vi "Store Configuration Parameters.vi"(8 "error in (no error)":errorcluster, 10 "refnum":T1, 11 "VacuumLine Configuration in":refnum<class "VacuumLine Configuration.lvclass">) -> (0 "error out":errorcluster, 2 "refnum out":T1, 3 "VacuumLine Configuration out":refnum<class "VacuumLine Configuration.lvclass">)   [LabVIEW 2016, in "Hardware.lvlib" / "VacuumLine.lvlib" / "VacuumLine Configuration.lvclass"]
uses:
  <userlib>/Common Components/Hardware/Abstract System/VacuumLine/VacuumLine Config/VacuumLine Configuration.lvclass
  <vilib>/Utility/config.llb/Config Data RefNum.ctl
  <userlib>/Common Components/Hardware/Abstract System/VacuumLine/VacuumLine Config/VacuumLine Configuration.lvclass/VacuumLine Configuration.ctl
  <userlib>/Common Components/Hardware/Abstract System/VacuumLine/VacuumLine/VacuumLine.lvclass/VacuumLine.ctl
  <userlib>/Common Components/Hardware/Abstract System/VacuumLine/VacuumLine/Read VacuumLine Params.vi
  <userlib>/Common Components/Hardware/Abstract System/VacuumLine/VacuumLine/Read Array of Move Button Configurations.vi
  <userlib>/Configuration Dialog Actor/Configuration.lvclass
  <userlib>/Common Components/Hardware/Motor/Motor Config/Motor Configuration.lvclass
  <vilib>/Utility/config.llb/NI_LVConfig.lvlib
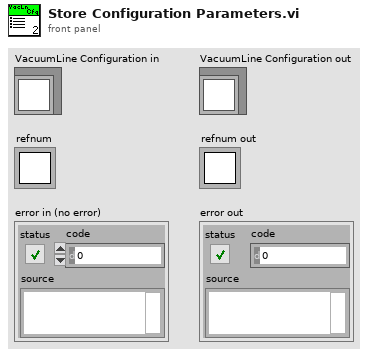
[diagram p1: front panel]
types:
  T1 = typedef "NI_LVConfig.lvlib/Config Data RefNum.ctl" = refnum<k1>
  T2 = typedef "Hardware.lvlib/VacuumLine.lvlib/VacuumLine.lvclass/VacuumLine Params.ctl" = cluster{"Motion Limits":cluster{"min":dbl, "max":dbl}, "No. of Conflict Zones":u8, "Conflict Zones (mm)":cluster{"with":string, "from":dbl, "to":dbl, "buffer":dbl}[], "Valve Complexes":T3[], "max( |Motor Pos - LRF Distance| )":dbl}
  T3 = typedef "Hardware.lvlib/VacuumLine.lvlib/VacuumLine.lvclass/Valve Complex.ctl" = cluster{"LogicIO Module":string, "Valve Open":T4, "Optical Switch -":T4, "Optical Switch +":T4, "Valve Closed Status Alert":cluster{"Pin#":u8, "Option":enum16{"Not Used", "Normally Closed"}}}
  T4 = typedef "Hardware.lvlib/VacuumLine.lvlib/VacuumLine.lvclass/Logic Cluster.ctl" = cluster{"Pin#":u8, "Location":dbl, "Tolerance":dbl}
  T5 = typedef "Hardware.lvlib/VacuumLine.lvlib/VacuumLine.lvclass/Button Config Cluster.ctl" = cluster{"Enabled?":bool, "Text on button":string, "Target pos":dbl}
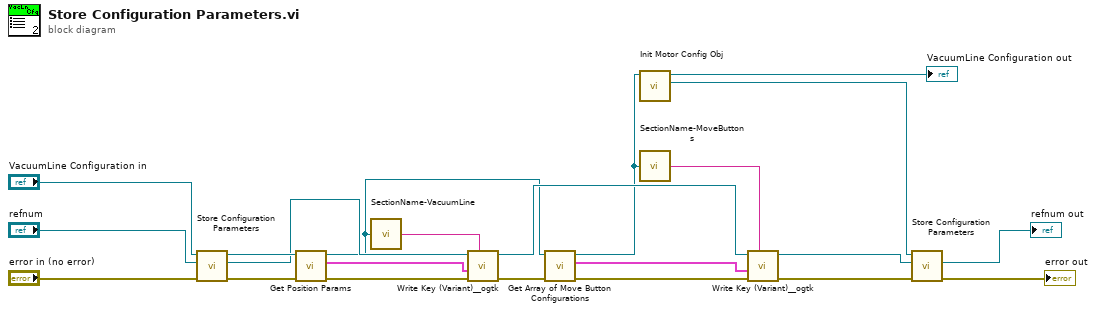
[diagram p0: block diagram]
diagram:
  n1 = call-parent "Store Configuration Parameters.vi"("error in (no error)"="error in (no error)", "refnum"="refnum", "Configuration in"="VacuumLine Configuration in") -> ("error out"=w22:errorcluster, "refnum out"=w17:T1, "Configuration out"=w18:refnum<class "VacuumLine Configuration.lvclass">)  [unwired: 6 in]
  n2 = call <userlib>:"Get Position Params.vi"("error in (no error)"=w22, "VacuumLine Configuration in"=w18) -> ("error out"=w9:errorcluster, "Position Params"=w16:T2, "VacuumLine Configuration out"=w3:refnum<class "VacuumLine Configuration.lvclass">)  [unwired: 7 in]
  n3 = call <userlib>:"SectionName-VacuumLine.vi"("VacuumLine Configuration in"=w3) -> ("SectionName"=w12:string)
  n4 = call <userlib>:"Write Key (Variant)__ogtk.vi"("section"=w12, "error in (no error)"=w9, "key-value"=w16, "refnum"=w17) -> ("error out"=w14:errorcluster, "refnum out"=w7:T1)  [unwired: 6 in]
  n5 = call <userlib>:"Get Array of Move Button Configurations.vi"("error in (no error)"=w14, "VacuumLine Configuration in"=w3) -> ("error out"=w4:errorcluster, "Array of Move Button Configurations"=w1:T5[], "VacuumLine Configuration out"=w2:refnum<class "VacuumLine Configuration.lvclass">)  [unwired: 7 in]
  n6 = call <userlib>:"Init Motor Config Obj.vi"("VacuumLine Configuration in"=w2) -> ("Motor Config Obj"=w10:refnum<class "Motor Configuration.lvclass">, "VacuumLine Configuration out"=→"VacuumLine Configuration out":refnum<class "VacuumLine Configuration.lvclass">)  [unwired: 8 in, 1 out]
  n7 = call <userlib>:"SectionName-MoveButtons.vi"("VacuumLine Configuration in"=w2) -> ("SectionName"=w5:string)
  n8 = call <userlib>:"Write Key (Variant)__ogtk.vi"("section"=w5, "error in (no error)"=w4, "key-value"=w1, "refnum"=w7) -> ("error out"=w8:errorcluster, "refnum out"=w6:T1)  [unwired: 6 in]
  n9 = call-dynamic "Store Configuration Parameters.vi"("error in (no error)"=w8, "refnum"=w6, "Example Configuration Dialog in"=w10) -> ("error out"=→"error out":errorcluster, "refnum out"=→"refnum out":T1)  [unwired: 6 in, 1 out]
